vi "Get Plugin Project and lvlibs.vi"(8 "error in":errorcluster, 10 "Custom Device name":string, 11 "CDEW_MetaDataObj in":refnum<class "NIVS_CDEW_MetaDataObj.lvclass">) -> (0 "error out":errorcluster, 3 "CDEW_MetaDataObj out":refnum<class "NIVS_CDEW_MetaDataObj.lvclass">)   [LabVIEW 2026, in "NIVS_CDEW_MetaDataObj.lvclass"]
uses:
  NIVS_CDEW_MetaDataObj.lvclass
  NIVS_CDEW_MetaDataObj.lvclass/NIVS_CDEW_MetaDataObj.ctl
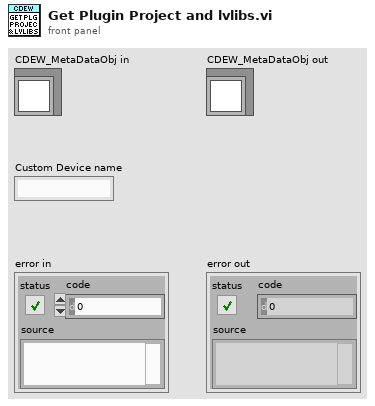
[diagram p1: front panel]
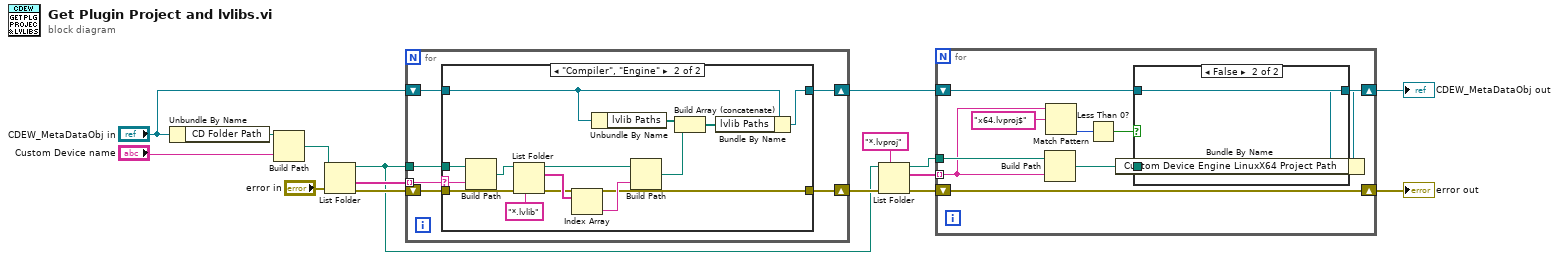
[diagram p0: block diagram]
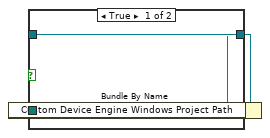
[diagram p2: hidden frame]
diagram:
  n1 = Unbundle By Name("CDEW_MetaDataObj in") -> ("CD Folder Path"=w11:path)
  n2 = Build Path(base path=w11, name or relative path="Custom Device name") -> (appended path=w12:path)
  n3 = List Folder(path=w12, error in="error in") -> (path out=w1:path, folder names=w15:string[], error out=w14:errorcluster)  [unwired: 2 in, 1 out]
  n4 = for {
    tunnel: w15 -> [w22] mode=indexing
    tunnel: w1 -> [w21]
    shift-right: [w19] -> w3
    shift-left: w14 -> [w20]
    shift-right: [w17] -> w9
    shift-left: "CDEW_MetaDataObj in" -> [w18]
    n5 = case shown="\"Compiler\", \"Engine\"" w22 {
      selector: w22 -> [_ w38]
      tunnel: w21 -> [_ w36]
      tunnel: w20 -> [w24 w31]
      tunnel: [w24 w30] -> w19
      tunnel: w18 -> [w23 w27]
      tunnel: [w23 w25] -> w17
      frame "False", Default {
      }
      frame "Compiler", "Engine" {
        n6 = Build Path(base path=w36, name or relative path=w38) -> (appended path=w37:path)
        n7 = List Folder(path=w37, pattern="*.lvlib", error in=w31) -> (path out=w33:path, filenames=w34:string[], error out=w30:errorcluster)  [unwired: 1 in, 1 out]
        n8 = Index Array(array=w34) -> (element=w32:string)  [unwired: 1 in]
        n9 = Unbundle By Name(w27) -> ("lvlib Paths"=w29:path[])
        n10 = Build Path(base path=w33, name or relative path=w32) -> (appended path=w28:path)
        n11 = Build Array (concatenate)(w29, w28) -> (w26:path[])
        n12 = Bundle By Name(cluster=w27, "lvlib Paths"=w26) -> (w25:refnum<class "NIVS_CDEW_MetaDataObj.lvclass">)
      }
    }
  }
  n13 = List Folder(path=w1, pattern="*.lvproj", error in=w3) -> (path out=w6:path, filenames=w5:string[], error out=w2:errorcluster)  [unwired: 1 in, 1 out]
  n14 = for {
    shift-right: [w39] -> w7
    shift-left: w9 -> [w42]
    shift-right: [w47] -> w8
    shift-left: w2 -> [w47]
    tunnel: w6 -> [w46]
    tunnel: w5 -> [w45] mode=indexing
    n15 = Build Path(base path=w46, name or relative path=w45) -> (appended path=w40:path)
    n16 = Match Pattern(string=w45, regular expression="x64.lvproj$") -> (offset past match=w43:i32)  [unwired: 1 in, 3 out]
    n17 = Less Than 0?(x=w43) -> (x < 0?=w41:bool)
    n18 = case shown="False" w41 {
      tunnel: w42 -> [w50 w53]
      tunnel: w40 -> [w49 w52]
      tunnel: [w48 w51] -> w39
      frame True {
        n19 = Bundle By Name(cluster=w50, "Custom Device Engine Windows Project Path"=w49) -> (w48:refnum<class "NIVS_CDEW_MetaDataObj.lvclass">)
      }
      frame False {
        n20 = Bundle By Name(cluster=w53, "Custom Device Engine LinuxX64 Project Path"=w52) -> (w51:refnum<class "NIVS_CDEW_MetaDataObj.lvclass">)
      }
    }
  }
  "error out" <- w8
  "CDEW_MetaDataObj out" <- w7
